vi "String-SelectAllText.vi"(8 "error in (no error)":errorcluster, 11 "String control ref":refnum<vi>) -> (0 "error out":errorcluster, 3 "reference out":refnum<vi>)   [LabVIEW 2020]
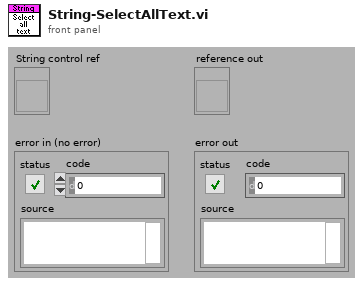
[diagram p1: front panel]
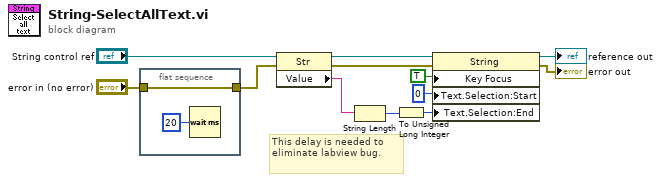
[diagram p0: block diagram]
diagram:
  # "This delay is needed to eliminate labview bug."
  n1 = flat-sequence {
    tunnel: [w13] -> w1
    tunnel: "error in (no error)" -> [w13]
    frame #0 {
      n2 = Wait (ms)(milliseconds to wait=u32 20) -> ()  [unwired: 1 out]
    }
  }
  n3 = property on="Property Node" class="Str"(reference="String control ref", error in=w1) -> (reference out=w7:refnum<vi>, error out=w5:errorcluster, "Value"=w8:string)
  n4 = String Length(string=w8) -> (length=w10:i32)
  n5 = To Unsigned Long Integer(number=w10) -> (unsigned 32bit integer=w6:u32)
  n6 = property on="Property Node" class="String"(reference=w7, error in=w5, "Key Focus"=TRUE, "Text.Selection:Start"=u32 0, "Text.Selection:End"=w6) -> (reference out=→"reference out":refnum<vi>, error out=→"error out":errorcluster)
